vi "Init Panel.vi"(8 "error in (no error)":errorcluster, 11 "vi reference":refnum<vi>) -> (0 "error out":errorcluster, 3 "vi reference (out)":refnum<vi>)   [LabVIEW 2020, in "WebServiceImporter.lvlib" / "Main Panel.lvlib"]
uses:
  <vilib>/Platform/WebService/Main Panel/Main Panel.lvlib
  <vilib>/Utility/miscctls.llb/LVPointTypeDef.ctl
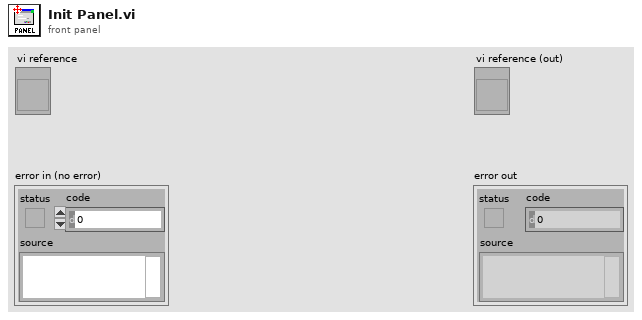
[diagram p1: front panel]
types:
  T1 = typedef "LVPointTypeDef.ctl" = cluster{"Horizontal":i16, "Vertical":i16}
  T2 = typedef "LVRectTypeDef.ctl" = cluster{"Left":i16, "Top":i16, "Right":i16, "Bottom":i16}
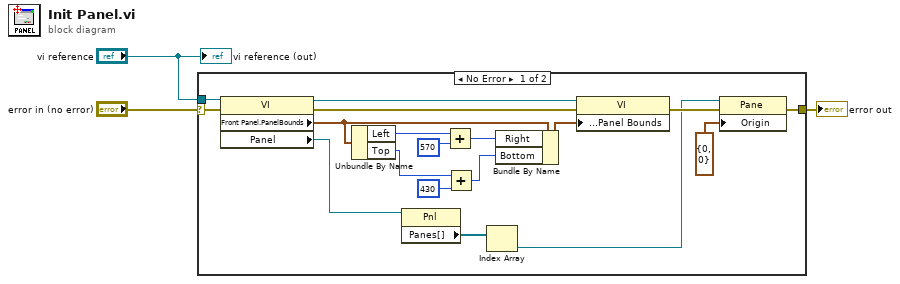
[diagram p0: block diagram]
diagram:
  n1 = case shown="No Error" "error in (no error)" {
    selector: "error in (no error)" -> [w20 w22]
    tunnel: "vi reference" -> [w21 _]
    tunnel: [w6 w22] -> w2
    frame No Error {
      n2 = property class="VI"(reference=w21, error in=w20) -> (reference out=w12:refnum<vi>, error out=w11:errorcluster, "Front Panel.PanelBounds"=w19:T2, "Panel"=w8:refnum<vi>)
      n3 = Unbundle By Name(w19) -> ("Left"=w18:i16, "Top"=w15:i16)
      n4 = property class="Pnl"(reference=w8) -> ("Panes[]"=w7:refnum<vi>[])  [unwired: 1 in, 2 out]
      n5 = Add(x=w18, y=i16 570) -> (x+y=w16:i16)
      n6 = Add(x=w15, y=i16 430) -> (x+y=w13:i16)
      n7 = Index Array(array=w7) -> (element=w5:refnum<vi>)  [unwired: 1 in]
      n8 = Bundle By Name(cluster=w19, "Right"=w16, "Bottom"=w13) -> (w9:T2)
      n9 = property class="VI"(reference=w12, error in=w11, "Front Panel Window:Panel Bounds"=w9) -> (error out=w10:errorcluster)  [unwired: 1 out]
      n10 = property class="Pane"(reference=w5, error in=w10, "Origin"=T1 {"Horizontal"=0, "Vertical"=0}) -> (error out=w6:errorcluster)  [unwired: 1 out]
    }
    frame Error {
    }
  }
  "error out" <- w2
  "vi reference (out)" <- "vi reference"
